vi "Create Connection List.vi"(11 "Connection Pairs":T1(array[cluster])) -> (3 "Connection List":string)   [LabVIEW 2020, in "slsc-switch-benchmarks.lvlib"]
uses:
  slsc-switch-benchmarks.lvlib
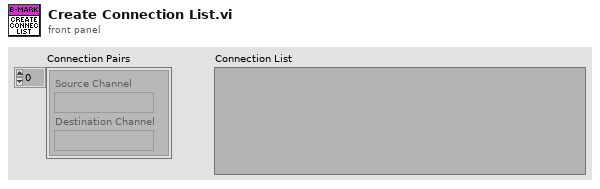
[diagram p1: front panel]
types:
  T1 = cluster{"Source Channel":string, "Destination Channel":string}[]
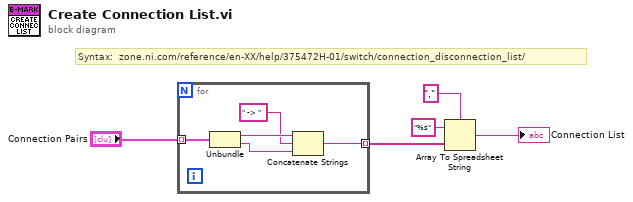
[diagram p0: block diagram]
diagram:
  # "Syntax:  zone.ni.com/reference/en-XX/help/375472H-01/switch/connection_disconnection_list/"
  n1 = for {
    tunnel: "Connection Pairs" -> [w10] mode=indexing
    tunnel: [w6] -> w4 mode=indexing
    n2 = Unbundle(w10) -> ("Source Channel"=w9:string, "Destination Channel"=w8:string)
    n3 = Concatenate Strings(w9, " -> " ("string"), w8) -> (w6:string)
  }
  n4 = Array To Spreadsheet String(delimiter (Tab)=",", array=w4, 3:"%s" ("format string")) -> (spreadsheet string=→"Connection List":string)
